vi "NanotecSMCPDDriver.move relative.vi"(0 "VISA resource name":refnum<visa-resource-name>, 1 "contollerID":i32=-1, 3 "nOfSteps [uSteps]":i32, 5 "error in (no error)":errorcluster) -> (14 "VISA resource name out":refnum<visa-resource-name>, 15 "contollerID out":i32=-1, 19 "error out":errorcluster)   [LabVIEW 2015, in "NanotecSMCPDDriver.lvlib"]
doc: "Performs a relative movement to a requested position. When using this VI, the controller should be in state \"ready\". This VI just starts the movement. It does not wait until the final position is reached."
uses:
  NanotecSMCPDDriver.lvlib
  Private/NanotecSMCPDDriver.positioning mode types.ctl
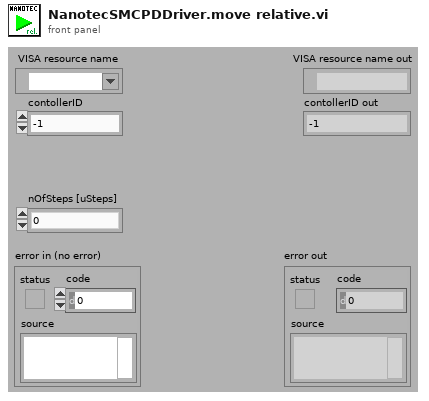
[diagram p1: front panel]
types:
  T1 = typedef "NanotecSMCPDDriver.lvlib/NanotecSMCPDDriver.positioning mode types.ctl" = enum16{"unknown", "relative positioning", "absolute positioning", "internal referencing", "external referencing"}
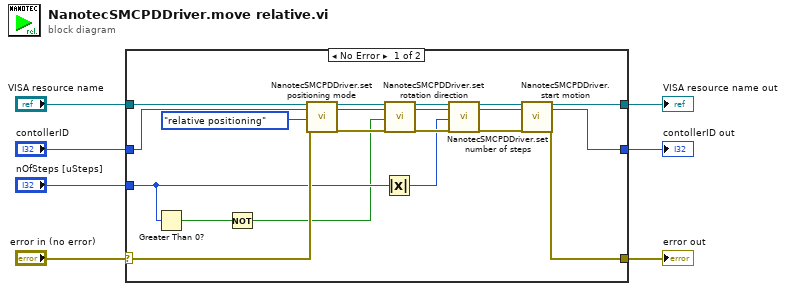
[diagram p0: block diagram]
diagram:
  n1 = case shown="No Error" "error in (no error)" {
    selector: "error in (no error)" -> [w20 w28]
    tunnel: [w25 w30] -> w7
    tunnel: [w21 w28] -> w6
    tunnel: "VISA resource name" -> [w27 w30]
    tunnel: "contollerID" -> [w24 w29]
    tunnel: [w22 w29] -> w3
    tunnel: "nOfSteps [uSteps]" -> [w11 _]
    frame No Error {
      n2 = Greater Than 0?(x=w11) -> (x > 0?=w9:bool)
      n3 = Not(x=w9) -> (.not. x?=w8:bool)
      n4 = call "NanotecSMCPDDriver.set positioning mode.vi"("VISA resource name"=w27, "contollerID"=w24, "positioningMode"=NanotecSMCPDDriver.positioning_mode_types."relative positioning", "error in (no error)"=w20) -> ("VISA resource name out"=w17:refnum<visa-resource-name>, "contollerID out"=w14:i32, "error out"=w13:errorcluster)  [unwired: 13 in]
      n5 = Absolute Value(x=w11) -> (abs(x)=w10:i32)
      n6 = call "NanotecSMCPDDriver.set rotation direction.vi"("VISA resource name"=w17, "contollerID"=w14, "clock-wise"=w8, "error in (no error)"=w13) -> ("VISA resource name out"=w16:refnum<visa-resource-name>, "contollerID out"=w15:i32, "error out"=w12:errorcluster)  [unwired: 13 in]
      n7 = call "NanotecSMCPDDriver.set number of steps.vi"("VISA resource name"=w16, "contollerID"=w15, "nOfSteps [uSteps]"=w10, "error in (no error)"=w12) -> ("VISA resource name out"=w26:refnum<visa-resource-name>, "contollerID out"=w23:i32, "error out"=w19:errorcluster)  [unwired: 13 in]
      n8 = call "NanotecSMCPDDriver.start motion.vi"("VISA resource name"=w26, "contollerID"=w23, "error in (no error)"=w19) -> ("VISA resource name out"=w25:refnum<visa-resource-name>, "contollerID out"=w22:i32, "error out"=w21:errorcluster)  [unwired: 14 in]
    }
    frame Error {
    }
  }
  "VISA resource name out" <- w7
  "error out" <- w6
  "contollerID out" <- w3
